vi "Start Read Action.vi"(7 "Disk":string, 8 "error in (no error)":errorcluster, 9 "Block Size":u64, 10 "Thread":i32, 11 "File Worker in":refnum<class "File Worker.lvclass">) -> (0 "error out":errorcluster, 3 "File Worker out":refnum<class "File Worker.lvclass">)   [LabVIEW 2025, in "File Worker.lvlib" / "File Worker.lvclass"]
uses:
  File Worker.lvclass
  C:/Program Files/National Instruments/LabVIEW 2025/vi.lib/ActorFramework/Actor/Actor.lvclass
  <vilib>/ActorFramework/Actor/Actor.lvclass/Actor.ctl
  File Worker.lvclass/File Worker.ctl
  Main/Main Messages/Handle Read Speed Msg/Handle Read Speed Msg.lvclass/Handle Read Speed Msg.ctl
  <vilib>/ActorFramework/Message Enqueuer/Message Enqueuer.lvclass/Message Enqueuer.ctl
  Main/Main Messages/Read Done Msg/Read Done Msg.lvclass/Read Done Msg.ctl
  <vilib>/ActorFramework/Message Enqueuer/Enqueue.vi
  Main/Main Messages/Handle Read Speed Msg/Handle Read Speed Msg.lvclass
  C:/Program Files/National Instruments/LabVIEW 2025/vi.lib/ActorFramework/Message/Message.lvclass
  Main/Main Messages/Read Done Msg/Read Done Msg.lvclass
  <vilib>/ActorFramework/Message Priority Queue/Priority Enqueue.vi
  <vilib>/ActorFramework/Actor/Actor.lvclass
  <vilib>/ptbypt/NI_PtbyPt.lvlib
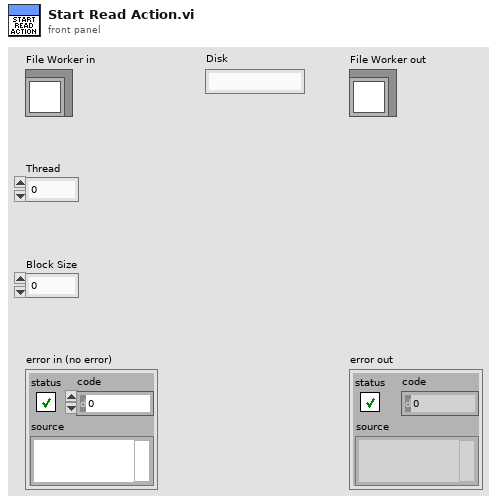
[diagram p1: front panel]
types:
  T1 = enum16{"open", "open or create", "create or replace", "create", "open (read-only)"}
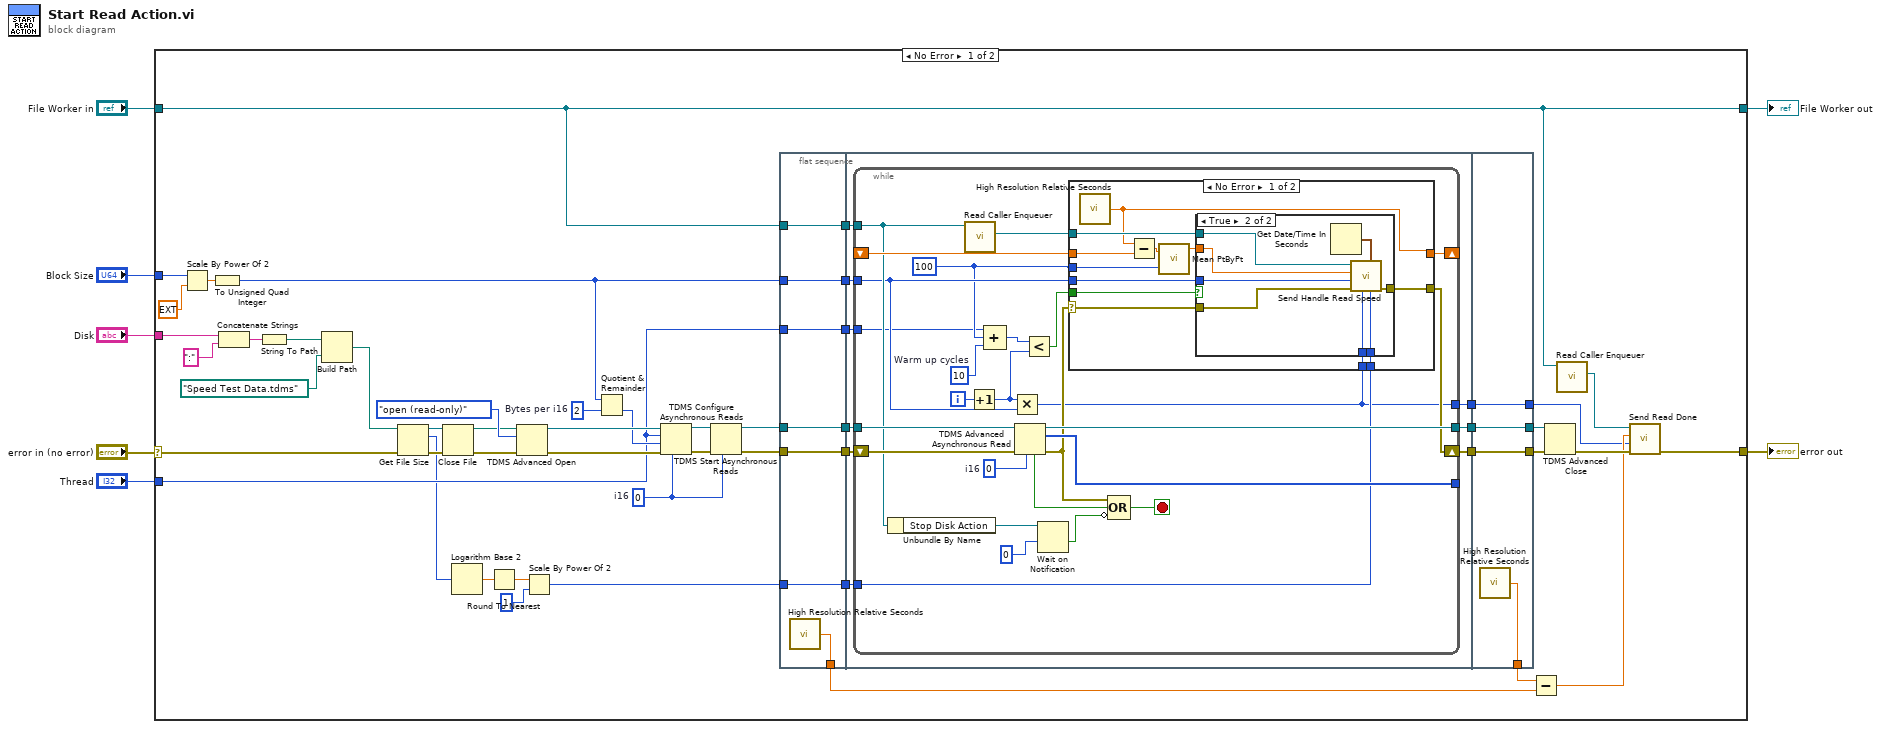
[diagram p0: block diagram]
diagram:
  n1 = case shown="No Error" "error in (no error)" {
    selector: "error in (no error)" -> [w15 w128]
    tunnel: [w26 w128] -> w6
    tunnel: [w28 w127] -> w4
    tunnel: "File Worker in" -> [w28 w127]
    tunnel: "Disk" -> [w41 _]
    tunnel: "Thread" -> [w20 _]
    tunnel: "Block Size" -> [w40 _]
    frame No Error {
      w46 = u64 2  # Bytes per i16
      w50 = i16 0  # i16
      n2 = Scale By Power Of 2(n=w40, x=ext 1.0) -> (x*2^n=w38:ext)
      n3 = To Unsigned Quad Integer(1:w38) -> (0:w37:u64)
      n4 = Concatenate Strings(w41, ":" ("string")) -> (w43:string)
      n5 = String To Path(string=w43) -> (path=w44:path)
      n6 = Build Path(base path=w44, name or relative path=path "Speed Test Data.tdms") -> (appended path=w19:path)
      n7 = Get File Size(file=w19, error in=w15) -> (refnum out=w18:refnum<file>, size (in bytes)=w13:i64, 0:w17:errorcluster)
      n8 = Close File(refnum=w18, error in=w17) -> (path=w16:path, error out=w14:errorcluster)
      n9 = Logarithm Base 2(1:w13) -> (0:w12:dbl)
      n10 = Round To Nearest(number=w12) -> (nearest integer value=w11:dbl)
      n11 = TDMS Advanced Open(8:w14, 10:T1."open (read-only)" ("Operation"), 11:w16) -> (0:w49:errorcluster, 3:w48:refnum<k34>)  [unwired: 2 in, 1 out]
      n12 = Scale By Power Of 2(n=w11, x=u64 1) -> (x*2^n=w9:u64)
      n13 = Quotient & Remainder(x=w37, y=w46) -> (floor(x/y)=w47:u64)  [unwired: 1 out]
      n14 = TDMS Configure Asynchronous Reads(6:w50, 8:w49, 9:w47, 10:w20, 11:w48) -> (0:w52:errorcluster, 3:w51:refnum<k34>)  [unwired: 1 in]
      n15 = TDMS Start Asynchronous Reads(6:w50, 8:w52, 11:w51) -> (0:w57:errorcluster, 3:w56:refnum<k34>)  [unwired: 1 in]
      n16 = flat-sequence {
        tunnel: w37 -> [w61]
        tunnel: w28 -> [w62]
        tunnel: w56 -> [w63]
        tunnel: w57 -> [w64]
        tunnel: [w64] -> w34
        tunnel: [w63] -> w33
        tunnel: [w62] -> w32
        tunnel: [w61] -> w31
        tunnel: [w60] -> w29
        tunnel: [w59] -> w21
        tunnel: w20 -> [w59]
        tunnel: w9 -> [w58]
        tunnel: [w58] -> w8
        tunnel: [w71] -> w36
        tunnel: [w70] -> w35
        tunnel: w34 -> [w73]
        tunnel: w33 -> [w72]
        tunnel: w32 -> [w69]
        tunnel: w31 -> [w68]
        tunnel: [w67] -> w22
        tunnel: w21 -> [w66]
        tunnel: w8 -> [w65]
        tunnel: [w125] -> w54
        tunnel: [w126] -> w55
        tunnel: w36 -> [w126]
        tunnel: w35 -> [w125]
        tunnel: [w124] -> w30
        tunnel: [w123] -> w23
        tunnel: w22 -> [w123]
        frame #0 {
          n17 = call <vilib>:"High Resolution Relative Seconds.vi"() -> ("relative seconds"=w60:dbl)
        }
        frame #1 {
          n18 = while {
            tunnel: [w98] -> w70
            shift-right: [w93] -> w71
            shift-left: w73 -> [w99]
            tunnel: w72 -> [w95]
            tunnel: [w97] -> _
            tunnel: w69 -> [w83]
            shift-right: [w90] -> _
            shift-left: _ -> [w89]
            tunnel: w68 -> [w80]
            tunnel: [w74] -> w67
            tunnel: w66 -> [w77]
            tunnel: w65 -> [w76]
            i -> [w81]
            stop <- w87 stop-if-true
            w78 = 100 ("Thread")
            w82 = 10  # Warm up cycles
            w96 = i16 0  # i16
            n19 = Unbundle By Name(w83) -> ("Stop Disk Action"=w85:refnum<notifier>)
            n20 = call <vilib>:"Read Caller Enqueuer.vi"("Actor"=w83) -> ("Caller Enqueuer"=w94:refnum<class "Message Enqueuer.lvclass">)  [unwired: 10 in]
            n21 = Increment(x=w81) -> (x+1=w75:i32)
            n22 = Compound Arithmetic op=unknown(w77, w78, w82) -> (w92:i32)
            n23 = Multiply(x=w75, y=w80) -> (x*y=w74:u64)
            n24 = TDMS Advanced Asynchronous Read(6:w96, 8:w99, 11:w95) -> (0:w86:errorcluster, 2:w97:i16[], 3:w98:refnum<k34>, 4:w88:bool)
            n25 = Less?(x=w92, y=w75) -> (x < y?=w91:bool)
            n26 = Wait on Notification(notifier=w85, timeout in ms (-1)=0) -> (timed out?=w79:bool)  [unwired: 2 in, 3 out]
            n27 = case shown="No Error" w86 {
              selector: w86 -> [w110 w122]
              tunnel: w94 -> [w111 _]
              tunnel: [w109 w122] -> w93
              tunnel: w91 -> [w108 _]
              tunnel: [w107 w121] -> w90
              tunnel: w89 -> [w106 w121]
              tunnel: w80 -> [w105 _]
              tunnel: w78 -> [w102 _]
              tunnel: w76 -> [w101 _]
              tunnel: w74 -> [w100 _]
              frame No Error {
                n28 = call <vilib>:"High Resolution Relative Seconds.vi"() -> ("relative seconds"=w107:dbl)
                n29 = Subtract(x=w107, y=w106) -> (x-y=w104:dbl)
                n30 = call <vilib>:"Mean PtByPt.vi"("x"=w104, "sample length"=w102) -> ("mean"=w103:dbl)  [unwired: 2 in, 1 out]
                n31 = case shown="True" w108 {
                  tunnel: w111 -> [_ w120]
                  tunnel: w110 -> [w112 w117]
                  tunnel: [w112 w116] -> w109
                  tunnel: w103 -> [_ w119]
                  tunnel: w105 -> [_ w118]
                  tunnel: w101 -> [_ w114]
                  tunnel: w100 -> [_ w113]
                  frame False {
                  }
                  frame True {
                    n32 = Get Date/Time In Seconds() -> (seconds since 1Jan1904=w115:timestamp)
                    n33 = call "Send Handle Read Speed.vi"("Total Bytes"=w114, "Time Stamp"=w115, "Bytes Done"=w113, "error in (no error)"=w117, "Size"=w118, "Time"=w119, "Message Enqueuer"=w120) -> ("error out"=w116:errorcluster)  [unwired: 3 in, 1 out]
                  }
                }
              }
              frame Error {
              }
            }
            n34 = Compound Arithmetic op=OR(w86, w88, invert w79) -> (w87:bool)
          }
        }
        frame #2 {
          n35 = call <vilib>:"High Resolution Relative Seconds.vi"() -> ("relative seconds"=w124:dbl)
        }
      }
      n36 = Subtract(x=w30, y=w29) -> (x-y=w24:dbl)
      n37 = TDMS Advanced Close(8:w55, 11:w54) -> (0:w27:errorcluster)  [unwired: 2 in, 1 out]
      n38 = call <vilib>:"Read Caller Enqueuer.vi"("Actor"=w28) -> ("Caller Enqueuer"=w25:refnum<class "Message Enqueuer.lvclass">)  [unwired: 10 in]
      n39 = call "Send Read Done.vi"("error in (no error)"=w27, "Bytes"=w23, "Time"=w24, "Message Enqueuer"=w25) -> ("error out"=w26:errorcluster)  [unwired: 6 in, 1 out]
    }
    frame Error {
    }
  }
  "error out" <- w6
  "File Worker out" <- w4
